vi "TestUI.vi"() -> ()   [LabVIEW 2017]
panel:
  out "System Intensity Chart":dbl[][](graph)
  in  "Tab Control":enum32{"Page 1", "Page 2"}(tab)
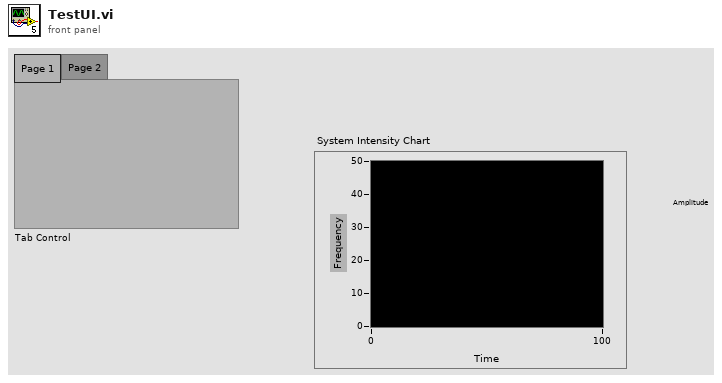
[diagram p1: front panel]
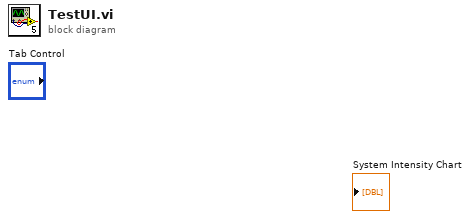
[diagram p0: block diagram]
diagram:
